vi "Pfeiffer Vacuum HLT5xx Special.vi"(8 "error in (no error)":errorcluster, 9 "PV HLT5xx Special - Cluster":T1={"Parameter"=0, "Parameter\nread only<->describe"=FALSE, "Anodenpotential Mass 2"=905, "Anodenpotential Mass 3"=610, "Anodenpotential Mass 4"=465, "Filament"=0, "Zero time [s]"=5} {"Zero time [s]" min=2 max=200 step=1; "Filament" items=["Emission off", "Kathode 1, Emission on", "Kathode 2, Emission on", "Emission on"]; "Anodenpotential Mass 4" min=390 max=520 step=1; "Anodenpotential Mass 3" min=510 max=610 step=1; "Anodenpotential Mass 2" min=785 max=995 step=1; "Parameter" items=[" Preamplifier voltage [mV] (read only)", " Anode voltage [V] (read only)", " Kathode voltage [V] (read only)", " Suppressor voltage [V] (read only)", " Anodenpotential Mass 2 [V]", " Anodenpotential Mass 3 [V]", " Anodenpotential Mass 4 [V]", " Filament", " Zero time [s]"]}, 10 "Adress of unit":u16=1 min=1 max=999 step=1, 11 "COM Port Name in":refnum<visa-resource-name>="COM1") -> (0 "error out":errorcluster, 3 "response (data)":string)   [LabVIEW 2021]
doc: "This VI is an example of how to use the Pfeiffer Vacuum subVIs programmatically. This VI first initializes the instrument, takes measurements, then closes the instrument."
uses:
  <instrlib>/Pfeiffer Vacuum/Public/LeakDetector/PV HLT5xx Special - Cluster.ctl
  <instrlib>/Pfeiffer Vacuum/Pfeiffer Vacuum.lvlib
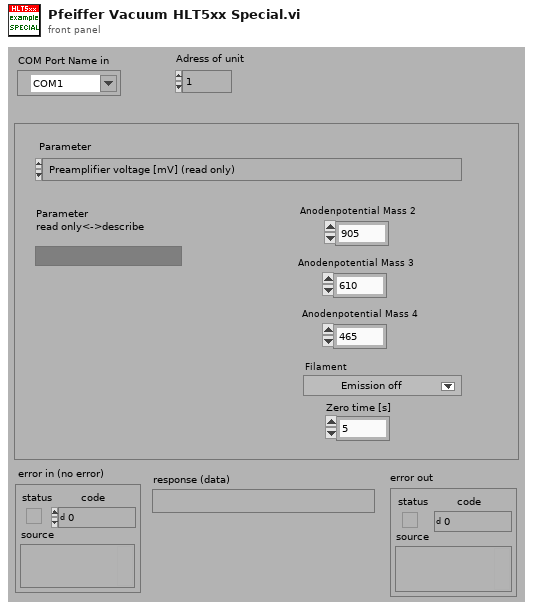
[diagram p1: front panel]
types:
  T1 = typedef "Pfeiffer Vacuum.lvlib/PV HLT5xx Special - Cluster.ctl" = cluster{"Parameter":u16, "Parameter\nread only<->describe":bool, "Anodenpotential Mass 2":u16, "Anodenpotential Mass 3":u16, "Anodenpotential Mass 4":u16, "Filament":u16, "Zero time [s]":u8}
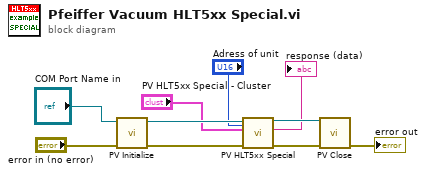
[diagram p0: block diagram]
diagram:
  n1 = call <instrlib>:"PV Initialize.vi"("error in (no error)"="error in (no error)", "VISA session in"="COM Port Name in") -> ("error out"=w10:errorcluster, "VISA session out"=w8:refnum<visa-resource-name>)  [unwired: 8 in]
  n2 = call <instrlib>:"PV HLT5xx Special.vi"("Adress of unit"="Adress of unit", "error in (no error)"=w10, "PV HLT5xx Special - Cluster"="PV HLT5xx Special - Cluster", "VISA session"=w8) -> ("error out"=w9:errorcluster, "response (data)"=→"response (data)":string, "dup VISA session"=w7:refnum<visa-resource-name>)  [unwired: 5 in]
  n3 = call <instrlib>:"PV Close.vi"("VISA session"=w7, "error in (no error)"=w9) -> ("error out"=→"error out":errorcluster)  [unwired: 13 in]
